vi "Available Maze Levels.vi"() -> (2 "Names":string[](array[string]), 3 "Available Mazes":refnum<class "MazeGen.lvclass">[](array[class]))   [LabVIEW 2020, in "Maze.lvlib" / "MazeGen.lvclass"]
uses:
  MazeGen.lvclass
  Intermediate MazeGen/Intermediate MazeGen.lvclass
  C:/dev/lv/2020/SoL/sol-maze/ProjectTemplates/Source/SummerOfLabVIEW/Summer of LabVIEW - Maze/template/Maze/MazeGen/MazeGen.lvclass
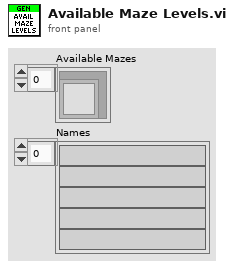
[diagram p1: front panel]
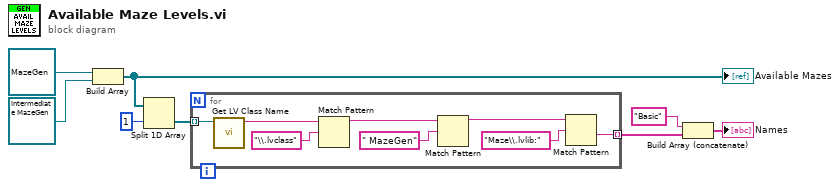
[diagram p0: block diagram]
diagram:
  n1 = Build Array(refnum<class "MazeGen.lvclass"> refnum ("Maze.lvlib:MazeGen.lvclass"), refnum<class "Intermediate MazeGen.lvclass"> refnum ("Maze.lvlib:Intermediate MazeGen.lvclass")) -> (w6:refnum<class "MazeGen.lvclass">[])
  "Available Mazes" <- w6
  n2 = Split 1D Array(array=w6, index=1) -> (second subarray=w7:refnum<class "MazeGen.lvclass">[])  [unwired: 1 out]
  n3 = for {
    tunnel: w7 -> [w16] mode=indexing
    tunnel: [w9] -> w4 mode=indexing
    n4 = call <vilib>:"Get LV Class Name.vi"("object"=w16) -> ("class name"=w15:string)  [unwired: 9 in, 1 out]
    n5 = Match Pattern(string=w15, regular expression="\\.lvclass") -> (before substring=w13:string)  [unwired: 1 in, 3 out]
    n6 = Match Pattern(string=w13, regular expression=" MazeGen") -> (before substring=w11:string)  [unwired: 1 in, 3 out]
    n7 = Match Pattern(string=w11, regular expression="Maze\\.lvlib:") -> (after substring=w9:string)  [unwired: 1 in, 3 out]
  }
  n8 = Build Array (concatenate)("Basic", w4) -> (→"Names":string[])
